vi "test lrs.vi"() -> ()   [LabVIEW 2014]
uses:
  <vilib>/Analysis/1siggen.llb/Ramp Pattern by Delta.vi
  Reusable/General/Math Utilities.lvlib
  <vilib>/Analysis/NI_AALBase.lvlib
panel:
  out "log2(x)":T1
  out "Waveform Graph":i16[](graph)
  out "DataOut":T2 {"Sf" format="%.2e"; "SII" format="%.0g"; "SfI" format="%.0g"; "Sft" format="%.2e"; "SI" format="%.2e"; "stI" format="%.0g"}
  in  "tau":dbl=65.0 format="%#_13g"
  in  "B":dbl format="%#_13g"
  in  "A":dbl=1.0 format="%#_13g"
  in  "end":dbl=1856.0 format="%#_13g"
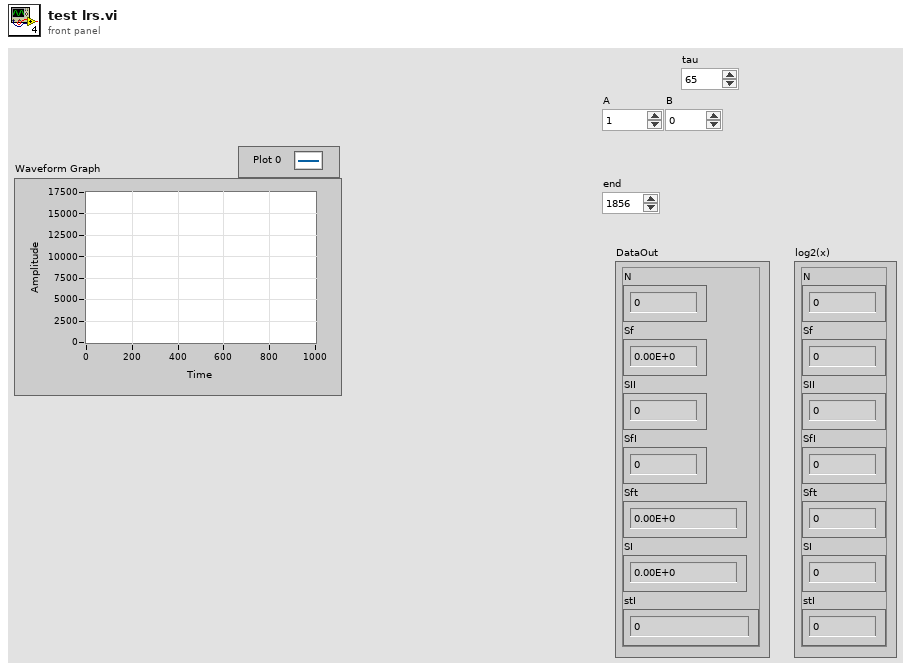
[diagram p1: front panel]
types:
  T1 = cluster{"N":dbl, "Sf":dbl, "SII":dbl, "SfI":dbl, "Sft":dbl, "SI":dbl, "stI":dbl}
  T2 = cluster{"N":i32, "Sf":fxp<+,54,54>, "SII":fxp<+,64,64>, "SfI":fxp<+,54,54>, "Sft":fxp<+,40,40>, "SI":fxp<+,54,54>, "stI":fxp<+,54,54>}
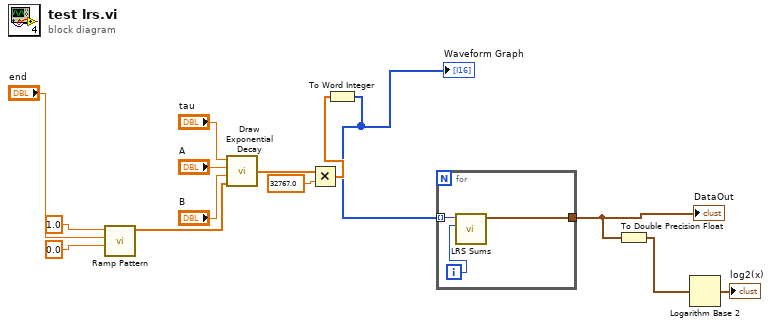
[diagram p0: block diagram]
diagram:
  n1 = call-poly <vilib>:"Ramp Pattern.vi"("start"=0.0, "end"="end", "delta"=1.0) -> ("Ramp Pattern"=w11:dbl[])  [unwired: 6 in, 2 out]
  n2 = call "Draw Exponential Decay.vi"("time"=w11, "B"="B", "A"="A", "tau"="tau") -> ("ExponentialOut"=w8:dbl[])
  n3 = Multiply(x=w8, y=32767.0) -> (x*y=w5:dbl[])
  n4 = To Word Integer(number=w5) -> (16bit integer=w4:i16[])
  "Waveform Graph" <- w4
  n5 = for {
    tunnel: w4 -> [w17] mode=indexing
    tunnel: [w15] -> w3
    i -> [w16]
    n6 = call "LRS Sums.vi"("i"=w16, "DataIn"=w17) -> ("DataOut"=w15:T2)  [unwired: 9 in]
  }
  "DataOut" <- w3
  n7 = To Double Precision Float(number=w3) -> (double precision float=w2:T1)
  n8 = Logarithm Base 2(1:w2) -> (0:→"log2(x)":T1)
